vi "Get XNET CAN Cluster List.vi"() -> (3 "XNET CAN Cluster List":string[](array[string]))   [LabVIEW 2021, in "Performanced XNET CAN Signal Logger.lvlib" / "Performanced XNET CAN Signal Logger.lvclass"]
uses:
  Performanced XNET CAN Signal Logger.lvclass
  Performanced XNET CAN Signal Logger.lvclass/Performanced XNET CAN Signal Logger.ctl
  <resource>/objmgr/xnet.rc
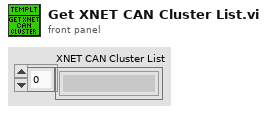
[diagram p1: front panel]
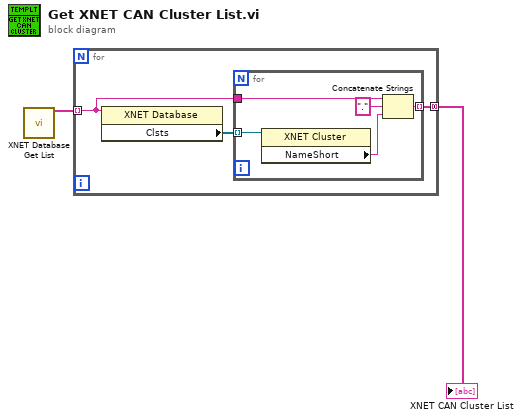
[diagram p0: block diagram]
diagram:
  n1 = call <vilib>:"XNET Database Get List.vi"() -> ("array of alias"=w1:string[])  [unwired: 13 in, 2 out]
  n2 = for {
    tunnel: w1 -> [w4] mode=indexing
    tunnel: [w3] -> w2 mode=concatenating
    n3 = property class="XNET Database"(reference=w4) -> ("Clsts"=w5:refnum<k21>[])  [unwired: 1 in, 2 out]
    n4 = for {
      tunnel: w5 -> [w10] mode=indexing
      tunnel: w4 -> [w9]
      tunnel: [w6] -> w3 mode=indexing
      n5 = property class="XNET Cluster"(reference=w10) -> ("NameShort"=w8:string)  [unwired: 1 in, 2 out]
      n6 = Concatenate Strings(w9, "." ("string"), w8) -> (w6:string)
    }
  }
  "XNET CAN Cluster List" <- w2
